vi "Set Debug Flags.vi"(10 "FIFO Debug Flags":refnum<class "Debug Flags FIFO.lvclass">, 11 "Pool in":refnum<class "Pool.lvclass">) -> (3 "Pool out":refnum<class "Pool.lvclass">)   [LabVIEW 2017, in "Data Sharing Framework Engine.lvlib" / "Pool.lvclass"]
uses:
  Pool.lvclass
  Debug/Debug Flags FIFO/Debug Flags FIFO.lvclass
  Pool.lvclass/Pool.ctl
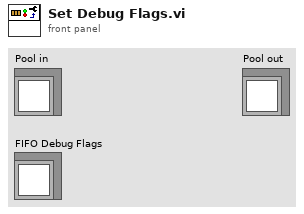
[diagram p1: front panel]
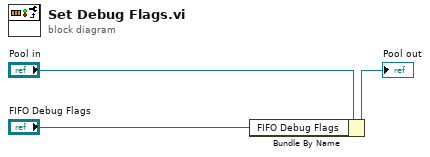
[diagram p0: block diagram]
diagram:
  n1 = Bundle By Name(cluster="Pool in", "FIFO Debug Flags"="FIFO Debug Flags") -> (→"Pool out":refnum<class "Pool.lvclass">)
